vi "collectFrame.vi"(7 "Reset":bool, 8 "error in (no error)":errorcluster, 10 "byte":u8, 11 "ASCII in":refnum<class "ASCII.lvclass">) -> (0 "error out":errorcluster, 1 "Data":i16[](array[numeric]), 2 "Finished":bool, 3 "ASCII out":refnum<class "ASCII.lvclass">, 5 "OK?":bool)   [LabVIEW 2017, in "ModBUS.lvlib" / "ASCII.lvclass"]
uses:
  ASCII.lvclass
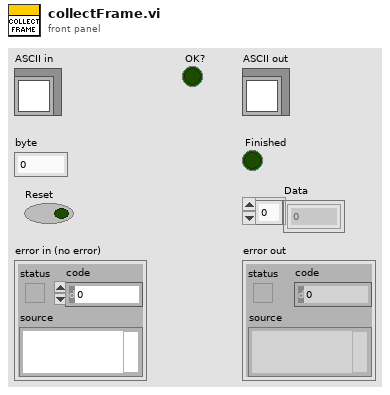
[diagram p1: front panel]
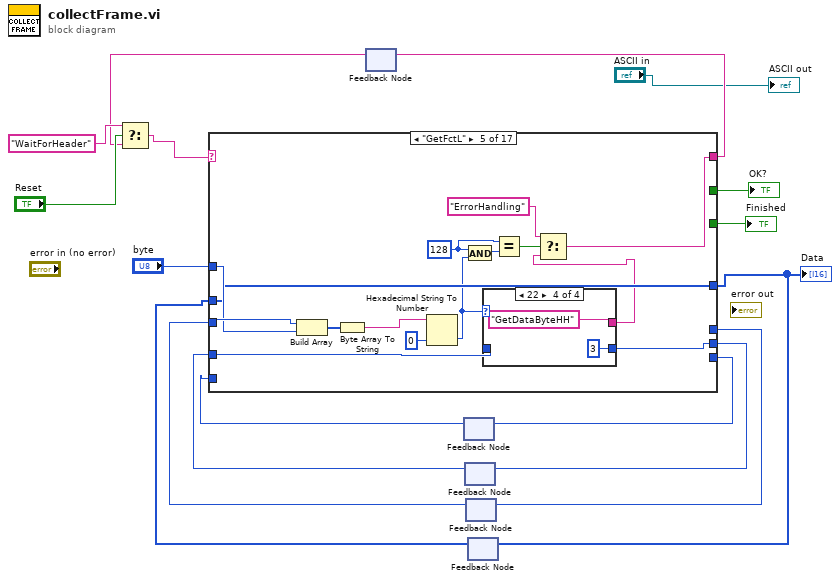
[diagram p0: block diagram]
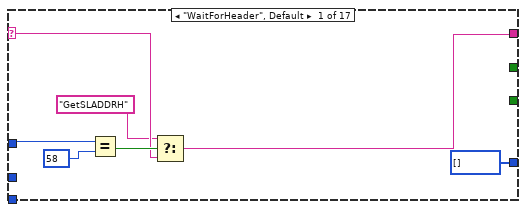
[diagram p2: hidden frame]
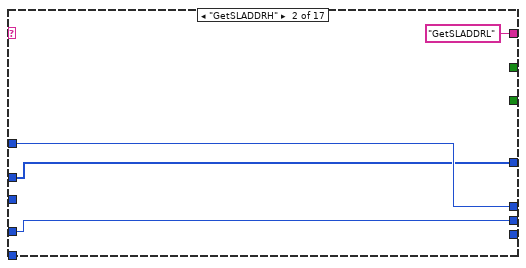
[diagram p3: hidden frame]
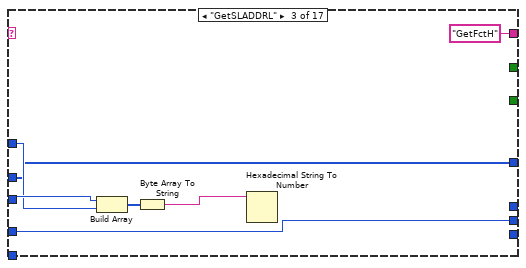
[diagram p4: hidden frame]
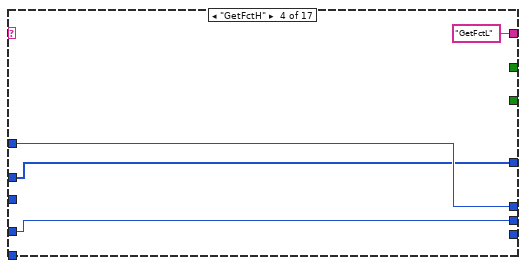
[diagram p5: hidden frame]
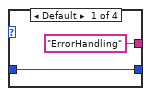
[diagram p6: hidden frame]
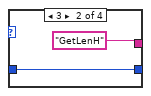
[diagram p7: hidden frame]
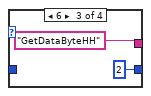
[diagram p8: hidden frame]
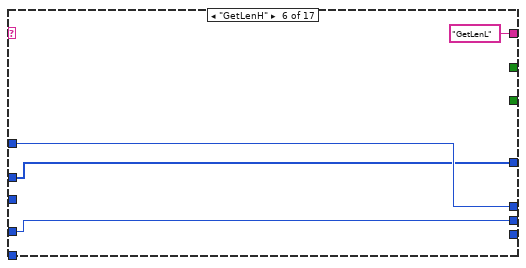
[diagram p9: hidden frame]
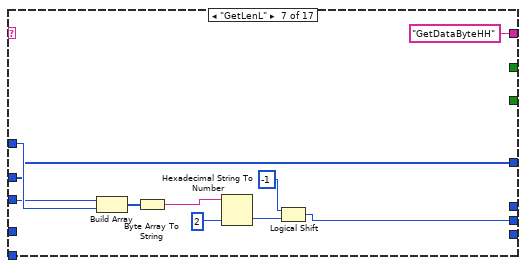
[diagram p10: hidden frame]
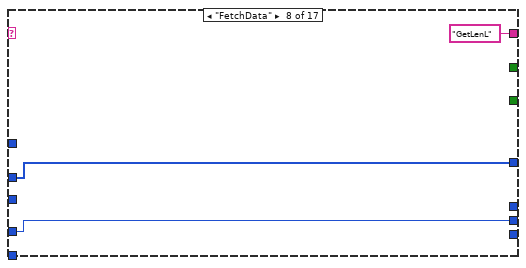
[diagram p11: hidden frame]
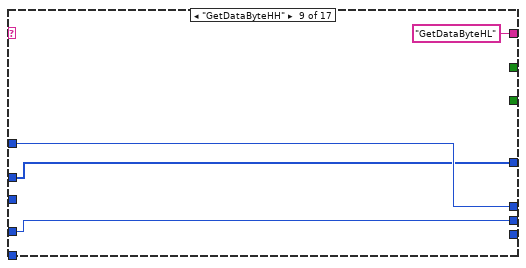
[diagram p12: hidden frame]
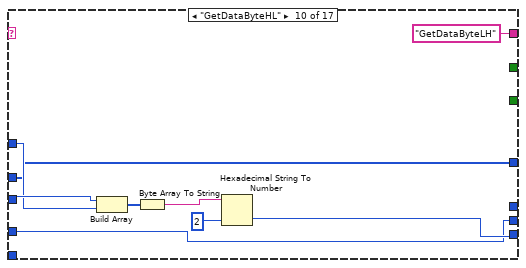
[diagram p13: hidden frame]
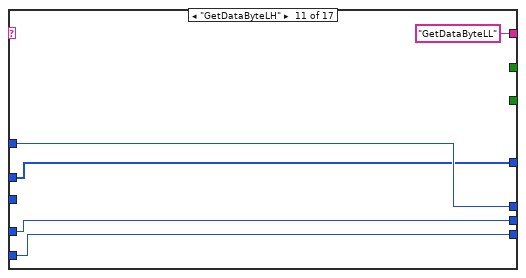
[diagram p14: hidden frame]
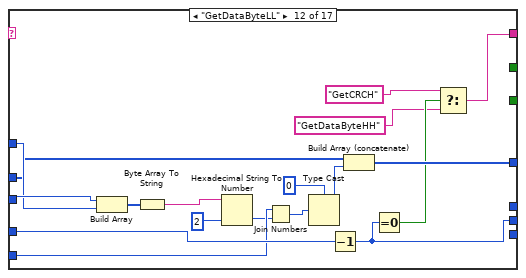
[diagram p15: hidden frame]
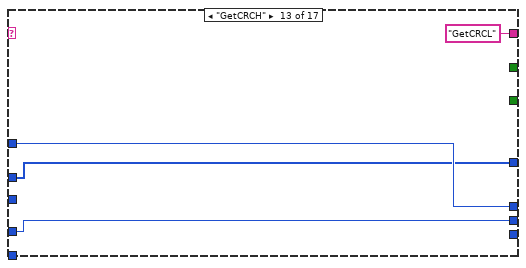
[diagram p16: hidden frame]
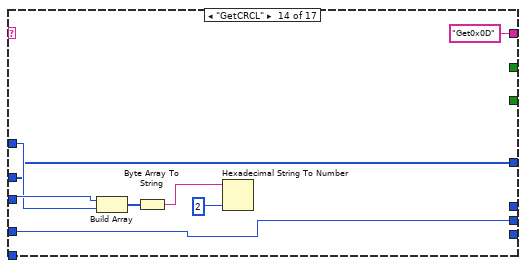
[diagram p17: hidden frame]
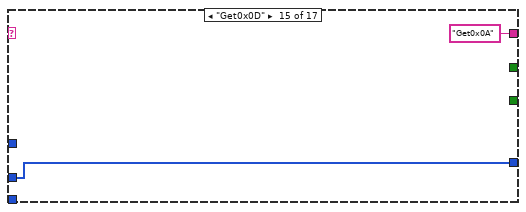
[diagram p18: hidden frame]
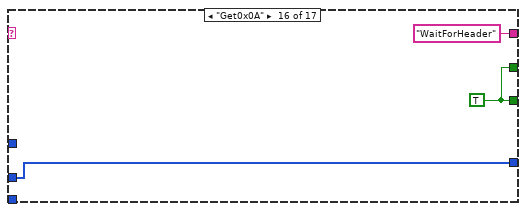
[diagram p19: hidden frame]
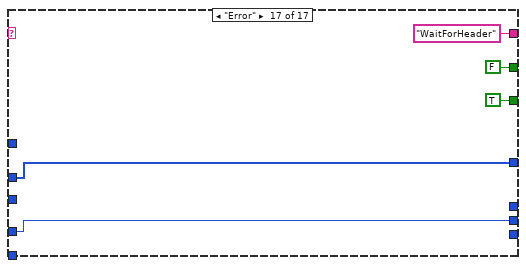
[diagram p20: hidden frame]
diagram:
  n1 = feedback #1() -> (w1:string)  [unwired: 1 in]
  n2 = Select(t="WaitForHeader", s="Reset", f=w1) -> (s? t:f=w3:string)
  n3 = feedback #2() -> (w10:u8)  [unwired: 1 in]
  n4 = feedback #3() -> (w12:u8)  [unwired: 1 in]
  n5 = feedback #4() -> (w14:u8)  [unwired: 1 in]
  n6 = feedback #5() -> (w8:i16[])  [unwired: 1 in]
  n7 = case shown="\"GetFctL\"" w3 {
    selector: w3 -> [w20 _ _ _ _ _ _ _ _ _ _ _ _ _ _ _ _]
    tunnel: [w21 "GetSLADDRL" ("t") "GetFctH" ("t") "GetFctL" ("t") w45 "GetLenL" ("t") "GetDataByteHH" ("t") "GetLenL" ("t") "GetDataByteHL" ("t") "GetDataByteLH" ("t") "GetDataByteLL" ("t") w98 "GetCRCL" ("t") "Get0x0D" ("t") "Get0x0A" ("t") "WaitForHeader" ("t") "WaitForHeader" ("t")] -> w17
    tunnel: "byte" -> [w24 w28 w34 w39 w53 w66 w76 _ w83 w91 w97 w114 w119 w126 _ _ _]
    tunnel: [_ w28 _ w39 _ w66 _ _ w83 _ w97 _ w119 _ _ _ _] -> w15
    tunnel: w14 -> [_ _ w35 _ w54 _ w67 _ _ w92 _ w115 _ w127 _ _ _]
    tunnel: [_ w26 w30 w37 w41 w64 w69 w78 w81 w85 w95 w102 w117 w120 _ _ w137] -> w13
    tunnel: w12 -> [_ w26 w30 w37 w40 w64 _ w78 w81 w85 w95 w110 w117 w120 _ _ w137]
    tunnel: [_ _ _ _ _ _ _ _ _ w86 w93 _ _ _ _ _ _] -> w11
    tunnel: w10 -> [_ _ _ _ _ _ _ _ _ _ w93 w109 _ _ _ _ _]
    tunnel: [i16[] [] w25 w29 w36 w44 w63 w68 w77 w80 w84 w94 w107 w116 w121 w128 w131 w136] -> w9
    tunnel: w8 -> [_ w25 w29 w36 w44 w63 w68 w77 w80 w84 w94 w106 w116 w121 w128 w131 w136]
    tunnel: [_ _ _ _ _ _ _ _ _ _ _ _ _ _ _ w130 TRUE ("Finished")] -> w7
    tunnel: [_ _ _ _ _ _ _ _ _ _ _ _ _ _ _ w130 FALSE ("Finished")] -> w5
    frame "WaitForHeader", Default {
      n8 = Equal?(x=w24, y=u8 58) -> (x = y?=w22:bool)
      n9 = Select(t="GetSLADDRH", s=w22, f=w20) -> (s? t:f=w21:string)
    }
    frame "GetSLADDRH" {
    }
    frame "GetSLADDRL" {
      n10 = Build Array(w35, w34) -> (w33:u8[])
      n11 = Byte Array To String(unsigned byte array=w33) -> (string=w32:string)
      n12 = Hexadecimal String To Number(string=w32) -> ()  [unwired: 2 in, 2 out]
    }
    frame "GetFctH" {
    }
    frame "GetFctL" {
      w48 = u8 128 ("x")
      n13 = Build Array(w54, w53) -> (w52:u8[])
      n14 = Byte Array To String(unsigned byte array=w52) -> (string=w51:string)
      n15 = Hexadecimal String To Number(string=w51, default (0uL)=u8 0 ("default (0 U32)")) -> (number=w43:u8)  [unwired: 1 in, 1 out]
      n16 = And(x=w48, y=w43) -> (x .and. y?=w49:u8)
      n17 = case shown="22" w43 {
        tunnel: ["ErrorHandling" ("t") "GetLenH" ("t") "GetDataByteHH" ("t") "GetDataByteHH" ("t")] -> w42
        tunnel: [w55 w57 u8 2 u8 3] -> w41
        tunnel: w40 -> [w55 w57 _ _]
        frame Default {
        }
        frame 3 {
        }
        frame 6 {
        }
        frame 22 {
        }
      }
      n18 = Equal?(x=w48, y=w49) -> (x = y?=w47:bool)
      n19 = Select(t="ErrorHandling", s=w47, f=w42) -> (s? t:f=w45:string)
    }
    frame "GetLenH" {
    }
    frame "GetLenL" {
      n20 = Build Array(w67, w76) -> (w75:u8[])
      n21 = Byte Array To String(unsigned byte array=w75) -> (string=w74:string)
      n22 = Hexadecimal String To Number(string=w74, default (0uL)=u8 2 ("y")) -> (number=w71:u8)  [unwired: 1 in, 1 out]
      n23 = Logical Shift(y=i16 -1, x=w71) -> (x << y=w69:u8)
    }
    frame "FetchData" {
    }
    frame "GetDataByteHH" {
    }
    frame "GetDataByteHL" {
      n24 = Build Array(w92, w91) -> (w90:u8[])
      n25 = Byte Array To String(unsigned byte array=w90) -> (string=w89:string)
      n26 = Hexadecimal String To Number(string=w89, default (0uL)=u8 2 ("y")) -> (number=w86:u8)  [unwired: 1 in, 1 out]
    }
    frame "GetDataByteLH" {
    }
    frame "GetDataByteLL" {
      n27 = Build Array(w115, w114) -> (w113:u8[])
      n28 = Byte Array To String(unsigned byte array=w113) -> (string=w112:string)
      n29 = Hexadecimal String To Number(string=w112, default (0uL)=u8 2 ("y")) -> (number=w108:u8)  [unwired: 1 in, 1 out]
      n30 = Join Numbers(hi=w109, lo=w108) -> ((hi.lo)=w105:u16)
      n31 = Type Cast(type=i16 0 ("(hi.lo)"), x=w105) -> (*(type *) &x=w104:i16)
      n32 = Decrement(x=w110) -> (x-1=w102:u8)
      n33 = Build Array (concatenate)(w106, w104) -> (w107:i16[])
      n34 = Equal To 0?(x=w102) -> (x = 0?=w101:bool)
      n35 = Select(t="GetCRCH", s=w101, f="GetDataByteHH" ("t")) -> (s? t:f=w98:string)
    }
    frame "GetCRCH" {
    }
    frame "GetCRCL" {
      n36 = Build Array(w127, w126) -> (w125:u8[])
      n37 = Byte Array To String(unsigned byte array=w125) -> (string=w124:string)
      n38 = Hexadecimal String To Number(string=w124, default (0uL)=u8 2 ("y")) -> ()  [unwired: 1 in, 2 out]
    }
    frame "Get0x0D" {
    }
    frame "Get0x0A" {
      w130 = TRUE ("Finished")
    }
    frame "Error" {
    }
  }
  "Data" <- w9
  "Finished" <- w7
  "OK?" <- w5
  n39 = feedback-in #1(w17) -> ()
  n40 = feedback-in #2(w11) -> ()
  n41 = feedback-in #3(w13) -> ()
  n42 = feedback-in #4(w15) -> ()
  n43 = feedback-in #5(w9) -> ()
  "ASCII out" <- "ASCII in"
